vi "merge_RS Bistable.vi"   [LabVIEW 2020, in "NI_FunctionBlockMergeVIs.lvlib"]
doc: "Creates a reset-dominant latch, also known as a flip-flop."
uses:
  <vilib>/functionblocks/NI_FunctionBlockMergeVIs.lvlib
  <vilib>/functionblocks/FB Core/FB Core.xnode
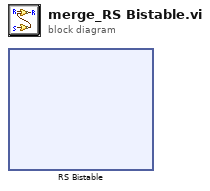
[diagram p0: block diagram]
diagram:
  n1 = xnode "RS Bistable"() -> ()  [unwired: 3 in, 2 out]
